vi "Network - Send PSP String.vi"(11 "Message":string) -> ()   [LabVIEW 2010]
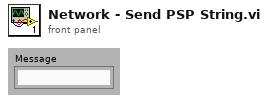
[diagram p1: front panel]
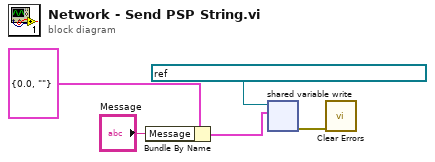
[diagram p0: block diagram]
diagram:
  n1 = Bundle By Name(cluster=cluster{"Channel":dbl, "Message":string} {"Channel"=0.0, "Message"=""}, "Message"="Message") -> (w3:cluster{"Channel":dbl, "Message":string})
  n2 = shared-variable-write(refnum<k21> "ni.var.psp://localhost/AcquisitionVariables/Message" ("shared variable refnum in"), w3) -> (w1:errorcluster)  [unwired: 1 in, 1 out]
  n3 = call <vilib>:"Clear Errors.vi"("error in (no error)"=w1) -> ()  [unwired: 6 in, 1 out]
